vi "WS2812(mycode).vi"() -> ()   [LabVIEW 2019]
uses:
  <vilib>/MakerHub/LINX/Public/Utilities/Open Serial.vi
  <vilib>/MakerHub/LINX/Public/Sensors/Lights/WS2812/Write N LEDs.vi
  <vilib>/ErrorRing/Error Ring.xnode
  <vilib>/MakerHub/LINX/Public/Sensors/Lights/WS2812/WS2812.lvlib
  <vilib>/MakerHub/LINX/LMH-LINX.lvlib
panel:
  in  "Serial Port":refnum<visa-resource-name>="N/A"
  in  "stop":bool
  in  "Colors":u32[](array[colorbox])
  in  "LED Index":u16
  in  "Number of LEDs":u16
  in  "Data Channel":u8
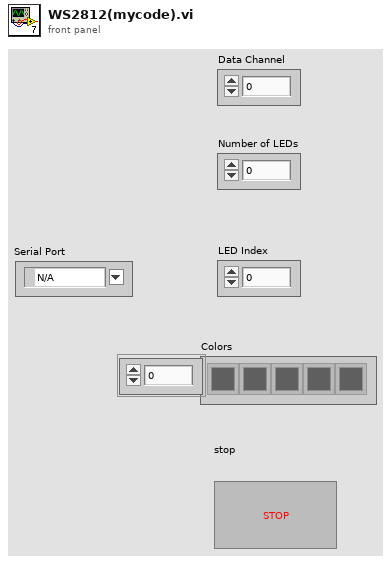
[diagram p1: front panel]
types:
  T1 = typedef "LMH-LINX.lvlib/LINX Ref.ctl" = cluster{"IO":T2, "Interface":T3, "LINX Device Config":T4}
  T2 = typedef "LMH-LINX.lvlib/Platform.ctl" = enum16{"Remote", "Local"}
  T3 = typedef "LMH-LINX.lvlib/Interface.ctl" = enum16{"Serial", "TCP"}
  T4 = typedef "LMH-LINX.lvlib/Device.lvlib/LINX Device Config.ctl" = cluster{"Interface":T3, "COM Port":refnum<visa-resource-name>, "TCP Configuration":T5, "Device Family":u8, "Device ID":u8, "Device Name":string, "TCP Ref":refnum<k5>, "Channels":T6}
  T5 = typedef "LMH-LINX.lvlib/Device.lvlib/TCP Config.ctl" = cluster{"IP Address":string, "Port":u16}
  T6 = typedef "LMH-LINX.lvlib/Channels.ctl" = cluster{"DI":u8[], "DO":u8[], "AI":u8[], "AO":u8[], "PWM":u8[], "QE":u8[], "UART":u8[], "I2C 2":u8[], "SPI":u8[], "CAN":u8[], "Servo":u8[], "AI Ref (V)":dbl, "AI Resolution (Bits)":u8, "AO Ref (V)":dbl, "AO Resolution (Bits)":u8}
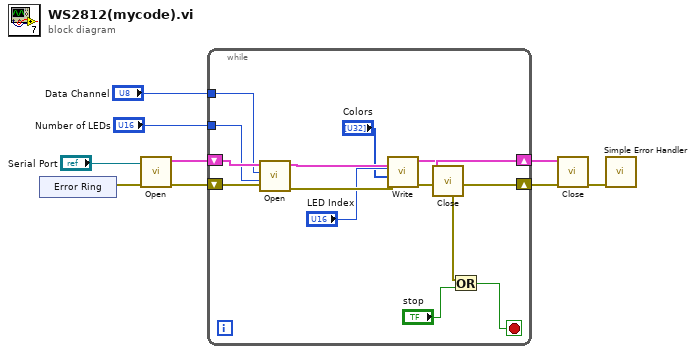
[diagram p0: block diagram]
diagram:
  n1 = xnode ("Error Ring")() -> ("error out"=w4:errorcluster)
  n2 = call-poly <vilib>:"Open.vi"("Error In"=w4, "Serial Port"="Serial Port") -> ("Error Out"=w5:errorcluster, "LINX Resource"=w6:T1)  [unwired: 7 in, 1 out]
  n3 = while {
    shift-right: [w10] -> w7
    shift-left: w5 -> [w18]
    shift-right: [w20] -> w8
    shift-left: w6 -> [w15]
    tunnel: "Data Channel" -> [w14]
    tunnel: "Number of LEDs" -> [w13]
    stop <- w11 stop-if-true
    n4 = call <vilib>:"Open.vi"("Error In"=w18, "Number of LEDs"=w13, "Data Channel"=w14, "LINX Resource"=w15) -> ("Error Out"=w19:errorcluster, "LINX Resource"=w21:T1)  [unwired: 6 in]
    n5 = call-poly <vilib>:"Write.vi"("Error In"=w19, "Colors"="Colors", "LED Index"="LED Index", "LINX Ref"=w21) -> ("Error Out"=w10:errorcluster, "LINX Ref"=w20:T1)  [unwired: 6 in]
    n6 = Or(x=w10, y="stop") -> (x .or. y?=w11:bool)
  }
  n7 = call <vilib>:"Close.vi"("Error In"=w7, "LINX Resource"=w8) -> ()  [unwired: 8 in, 2 out]
  n8 = call <vilib>:"Close.vi"("Error In"=w7, "LINX Resource"=w8) -> ("Error Out"=w9:errorcluster)  [unwired: 9 in]
  n9 = call <vilib>:"Simple Error Handler.vi"("error in (no error)"=w9) -> ()  [unwired: 4 in, 5 out]
